vi "GetAppName.vi"(8 "error in (no error)":errorcluster) -> (0 "error out":errorcluster, 3 "AppName":string)   [LabVIEW 2019, in "MicronServer.lvlib" / "ServiceBase.lvclass"]
uses:
  ServiceBase.lvclass
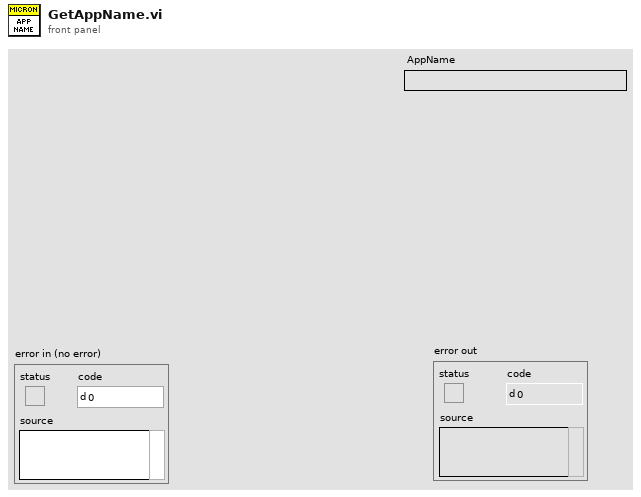
[diagram p1: front panel]
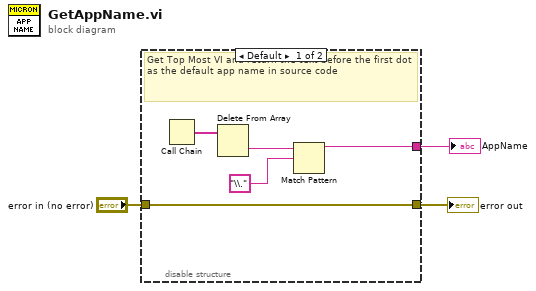
[diagram p0: block diagram]
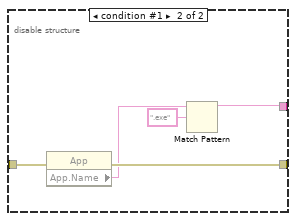
[diagram p2: hidden frame]
diagram:
  n1 = disable-structure shown="Default" {
    disable-tunnel: "error in (no error)" -> [w8 w13]
    disable-tunnel: [w8 w12] -> w2
    disable-tunnel: [w6 w9] -> w1
    frame condition #0 (active) {
      # "Get Top Most VI and return the text before the first dot as the default app name in source code"
      n2 = Call Chain() -> (call chain=w5:string[])
      n3 = Delete From Array(array=w5) -> (deleted portion=w4:string)  [unwired: 2 in, 1 out]
      n4 = Match Pattern(string=w4, regular expression="\\.") -> (before substring=w6:string)  [unwired: 1 in, 3 out]
    }
    frame condition #1 {
      n5 = property class="App"(error in=w13) -> (error out=w12:errorcluster, "App.Name"=w11:string)  [unwired: 1 in, 1 out]
      n6 = Match Pattern(string=w11, regular expression=".exe") -> (before substring=w9:string)  [unwired: 1 in, 3 out]
    }
  }
  "error out" <- w2
  "AppName" <- w1
